vi "Initialize.vi"(7 "UI Interaction":refnum<class "UI Interaction.lvclass">, 8 "error in (no error)":errorcluster {"code" format="Error %.0f"}, 10 "Settings Path":path, 11 "VIDoc Printer - Confluence In":refnum<class "VIDoc Printer - Confluence.lvclass">) -> (0 "error out":errorcluster {"code" format="Error %.0f"}, 3 "VIDoc Printer - Confluence Out":refnum<class "VIDoc Printer - Confluence.lvclass">)   [LabVIEW 2023, in "VIDoc Printer - Confluence.lvlib" / "VIDoc Printer - Confluence.lvclass"]
uses:
  VIDoc Printer - Confluence.lvclass
  UI Interaction/UI Interaction.lvclass
  <vilib>/Utility/sysdir.llb/System Directory Type.ctl
  VIDoc Printer - Confluence.lvclass/VIDoc Printer - Confluence.ctl
  Printer/VIDoc Printer.lvclass
  <userlib>/_PetranWay/LabVIEW Confluence API/Source/Confluence/Confluence Connection/Confluence.lvclass
  Settings/Confluence Printer Settings/VIDoc Settings - Confluence.lvclass
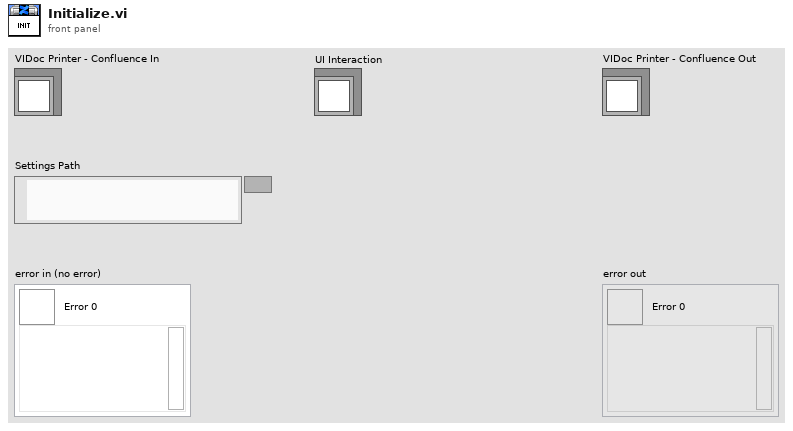
[diagram p1: front panel]
types:
  T1 = typedef "System Directory Type.ctl" = i32
  T2 = typedef "VIDoc Printer - Confluence.lvlib/VIDoc Settings - Confluence.lvclass/Confluence Printer Settings Cluster.ctl" = cluster{"Expand Structures":cluster{"VI Member":cluster{"By Folder Expand":bool, "By Tree Expand":bool, "By List Expand":bool, "Methods Expand":bool, "Controls Expand":bool}, "Control Member":cluster{"By Folder Expand":bool, "By Tree Expand":bool, "By List Expand":bool, "Controls Expand":bool}, "Interface":cluster{"List Expand":bool, "Controls Expand":bool, "Methods Expand":bool, "Inheritance Expand":bool}, "Library":cluster{"By Folder Expand":bool, "By Tree Expand":bool, "By List Expand":bool, "Controls Expand":bool, "Methods Expand":bool, "Inheritance Expand":bool}, "Class":cluster{"By Folder Expand":bool, "By Tree Expand":bool, "By List Expand":bool, "CPD Expand":bool, "Controls Expand":bool, "Methods Expand":bool, "Set Accessors Expand":bool, "Get Accessors Expand":bool, "Inheritance Expand":bool}}, "Sortable Tables":bool, "Table Column Ordering":cluster{"Class List":cluster{"Minimal":T3[], "Standard":T3[], "Full":T3[]}, "Library List":cluster{"Minimal":T3[], "Standard":T3[], "Full":T3[]}, "Control FP":cluster{"Minimal":T4[], "Standard":T4[], "Full":T4[]}, "Library Control Files":cluster{"Minimal":T5[], "Standard":T5[], "Full":T5[]}, "UI Methods":cluster{"Minimal":T5[], "Standard":T5[], "Full":T5[]}, "Method List":cluster{"Minimal":T5[], "Standard":T5[], "Full":T5[]}, "Interface Methods":cluster{"Minimal":T5[], "Standard":T5[], "Full":T5[]}, "LLB Methods":cluster{"Minimal":T5[], "Standard":T5[], "Full":T5[]}, "Library Methods":cluster{"Minimal":T5[], "Standard":T5[], "Full":T5[]}, "Class Methods":cluster{"Minimal":T5[], "Standard":T5[], "Full":T5[]}}}
  T3 = typedef "VIDoc Printer - Confluence.lvlib/VIDoc Settings - Confluence.lvclass/Class Info Column.ctl" = enum16{"Image", "Name", "Description", "Version", "Last Change", "Author", "Commit Hash", "Branch", "Qualified Name", "TransferMustOverrides", "ChildRefsRestricted"}
  T4 = typedef "VIDoc Printer - Confluence.lvlib/VIDoc Settings - Confluence.lvclass/Control Info Column.ctl" = enum16{"Image", "Name", "Description", "Caption", "Tip Strip", "Data Type", "Key Toggle"}
  T5 = typedef "VIDoc Printer - Confluence.lvlib/VIDoc Settings - Confluence.lvclass/VI Info Column.ctl" = enum16{"Name", "Conpane", "BD", "FP", "VI Icon", "Description", "Reentrant", "Inline", "Auto Error", "Compiled", "Code Complexity", "Data Size", "Debug", "Priority", "Rev", "Minimum Size", "Title", "FP Behavior", "FP Closeable", "Author", "Commit Hash", "Last Change", "Branch", "Scope", "Type", "Dispatch", "Must Override", "Must Use Parent", "Structure Tree"}
  T6 = typedef "VIDoc Printer - Confluence.lvlib/VIDoc Printer - Confluence.lvclass/Page Info.ctl" = cluster{"Page":refnum<class "Page.lvclass">, "Content":string, "Attachments":set{path}}
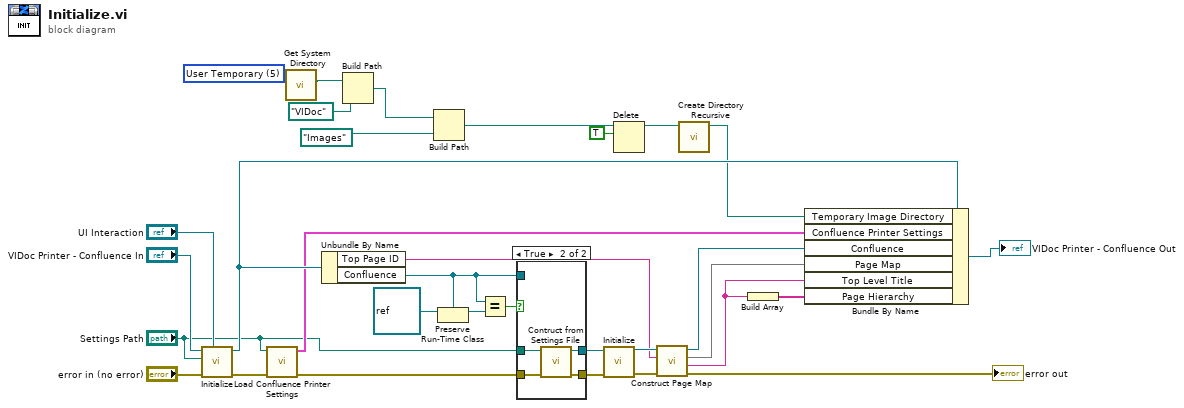
[diagram p0: block diagram]
diagram:
  w16 = T1 5 items=["User Home"=0, "User Desktop"=1, "User Documents"=2, "User Application Data"=3, "User Preferences"=4, "User Temporary"=5, "Public Documents"=6, "Public Application Data"=7, "Public Preferences"=8, "Public Cache"=13, "System Core Libraries"=9, "System Installed Libraries"=10, "Application Files"=11, "Boot Volume Root"=12] ("system directory type")
  n1 = call-parent "Initialize.vi"("UI Interaction"="UI Interaction", "error in (no error)"="error in (no error)", "Settings Path"="Settings Path", "VIDoc Printer In"="VIDoc Printer - Confluence In") -> ("error out"=w30:errorcluster, "VIDoc Printer Out"=w21:refnum<class "VIDoc Printer - Confluence.lvclass">)  [unwired: 6 in]
  n2 = call "Load Confluence Printer Settings.vi"("Error in"=w30, "Settings Path"="Settings Path") -> ("Error out"=w8:errorcluster, "Confluence Printer Settings"=w20:T2)  [unwired: 7 in, 1 out]
  n3 = call <vilib>:"Get System Directory.vi"("system directory type"=w16) -> ("system directory"=w17:path)  [unwired: 10 in]
  n4 = Unbundle By Name(w21) -> ("Top Page ID"=w26:string, "Confluence"=w1:refnum<class "Confluence.lvclass">)
  n5 = Build Path(base path=w17, name or relative path=path "VIDoc") -> (appended path=w15:path)
  n6 = Build Path(base path=w15, name or relative path=path "Images") -> (appended path=w12:path)
  n7 = Preserve Run-Time Class(object in=refnum<class> refnum, 2:w1) -> (object out=w2:refnum<class "Confluence.lvclass">)  [unwired: 1 in, 1 out]
  n8 = Equal?(x=w1, y=w2) -> (x = y?=w4:bool)
  n9 = case shown="True" w4 {
    tunnel: w8 -> [w33 w38]
    tunnel: "Settings Path" -> [_ w37]
    tunnel: [w34 w36] -> w6
    tunnel: [w33 w35] -> w5
    tunnel: w1 -> [w34 _]
    frame False {
    }
    frame True {
      n10 = call "Contruct from Settings File.vi"("Error in"=w38, "Settings Path"=w37) -> ("Error out"=w35:errorcluster, "Confluence out"=w36:refnum<class "Confluence.lvclass">)  [unwired: 8 in]
    }
  }
  n11 = call-dynamic "Initialize.vi"("Confluence in"=w6, "error in (no error)"=w5) -> ("Confluence out"=w29:refnum<class "Confluence.lvclass">, "error out"=w28:errorcluster)  [unwired: 12 in]
  n12 = Delete(path (use dialog)=w12, entire hierarchy (F)=TRUE) -> (deleted path=w11:path)  [unwired: 3 in, 2 out]
  n13 = call "Construct Page Map.vi"("error in (no error)"=w28, "Top Page ID"=w26, "Confluence Connection in"=w29) -> ("error out"=→"error out":errorcluster, "Top Page Title"=w10:string, "Page Map"=w24:map{string, T6}, "Confluence out"=w25:refnum<class "Confluence.lvclass">)  [unwired: 5 in]
  n14 = call <vilib>:"Create Directory Recursive.vi"("directory"=w11) -> ("directory copy"=w14:path)  [unwired: 4 in, 2 out]
  n15 = Build Array(w10) -> (w9:string[])
  n16 = Bundle By Name(cluster=w21, "Temporary Image Directory"=w14, "Confluence Printer Settings"=w20, "Confluence"=w25, "Page Map"=w24, "Top Level Title"=w10, "Page Hierarchy"=w9) -> (→"VIDoc Printer - Confluence Out":refnum<class "VIDoc Printer - Confluence.lvclass">)
